vi "CCD3000 Initialize.vi"(11 "Comm Params":T1={"Comm Interface"=1, "BUS"=0, "Address"=5, "Com Port"=1} {"Comm Interface" items=["RS 232", "GPIB"]}) -> (0 "error out":errorcluster, 3 "Success":bool)   [LabVIEW 2010]
uses:
  drivers/Horiba Spectrum One 3000V/Lib/CCD_command.llb/Comm Params.ctl
panel:
  in  "CCD ADC and Gain":dbl(ring) items=["16 bits Gain 1", "16 bits Gain 2", "16 bits Gain 3", "16 bits Gain 4", "14 bits Gain 1", "14 bits Gain 2"]
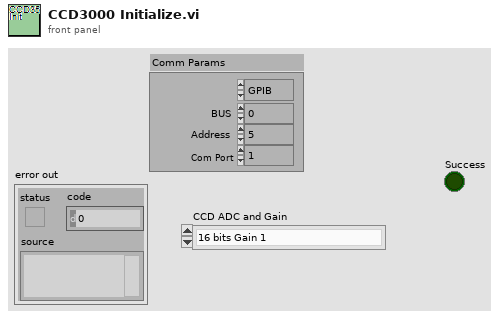
[diagram p1: front panel]
types:
  T1 = typedef "Comm Params.ctl" = cluster{"Comm Interface":u16, "BUS":i16, "Address":i16, "Com Port":i32}
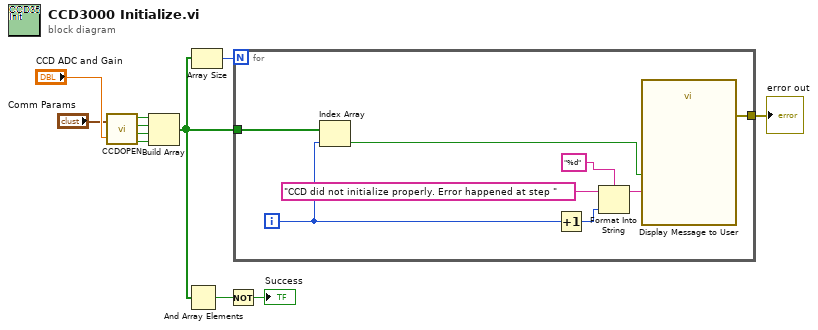
[diagram p0: block diagram]
diagram:
  n1 = call "CCDOPEN.VI"("CCD ADC and Gain"="CCD ADC and Gain", "Comm Params"="Comm Params") -> ("State Error"=w11:bool, "Table Error"=w10:bool, "Init Error"=w8:bool, "Boot Error"=w9:bool)  [unwired: 1 out]
  n2 = Build Array(w9, w8, w10, w11) -> (w5:bool[])
  n3 = And Array Elements(Boolean array=w5) -> (logical AND=w4:bool)
  n4 = Array Size(array=w5) -> (size(s)=w2:i32)
  n5 = Not(x=w4) -> (.not. x?=→"Success":bool)
  n6 = for {
    N: w2 -> [_]
    tunnel: w5 -> [w19]
    tunnel: [w12] -> w1
    i -> [w15]
    n7 = Index Array(array=w19, index=w15) -> (element=w18:bool)
    n8 = Increment(x=w15) -> (x+1=w14:i32)
    n9 = Format Into String(format string="%d", initial string="CCD did not initialize properly. Error happened at step ", w14) -> (resulting string=w13:string)  [unwired: 1 in, 1 out]
    n10 = call "Display Message to User"("Enable"=w18, "Message"=w13) -> ("error out"=w12:errorcluster)  [unwired: 8 in, 1 out]
  }
  "error out" <- w1
